vi "Set multiple channels.vi"(8 "values":dbl[](array[numeric]), 9 "names":string[](array[string]), 10 "Gateway IP Address (\"\": localhost)":string, 11 "Sequence Context":refnum<k7>) -> (0 "error out":errorcluster, 2 "Report Text":string)   [LabVIEW 2013, in "Set Channels.lvlib"]
uses:
  Set Channels.lvlib
  <vilib>/NI Veristand/Execution/Workspace/NI VeriStand - Set Multiple Channel Values.vi
  <vilib>/NI Veristand/Execution/Workspace/NI VeriStand - Get Multiple Channel Values.vi
  <vilib>/NI Veristand/Execution/Workspace/NI_VS Workspace ExecutionAPI.lvlib
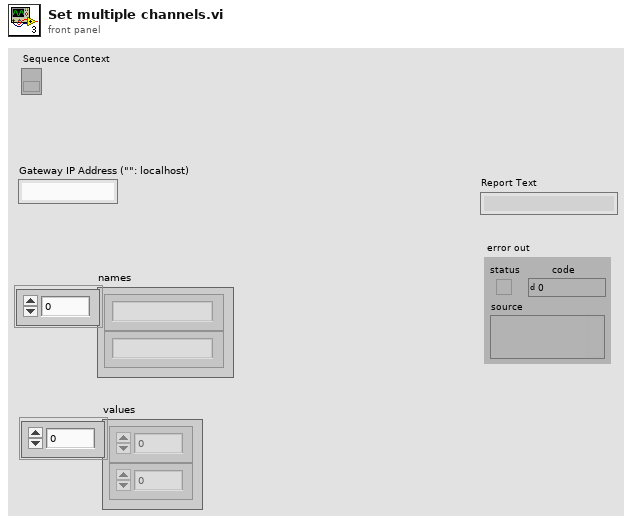
[diagram p1: front panel]
types:
  T1 = typedef "NI_VS Workspace ExecutionAPI.lvlib/WorkspaceAPI.ctl" = refnum<k24>
  T2 = typedef "TestStand - Status Monitor.ctl" = cluster{"Sequence Context":refnum<k7>, "Execution":refnum<k7>, "Termination Monitor":refnum<k7>}
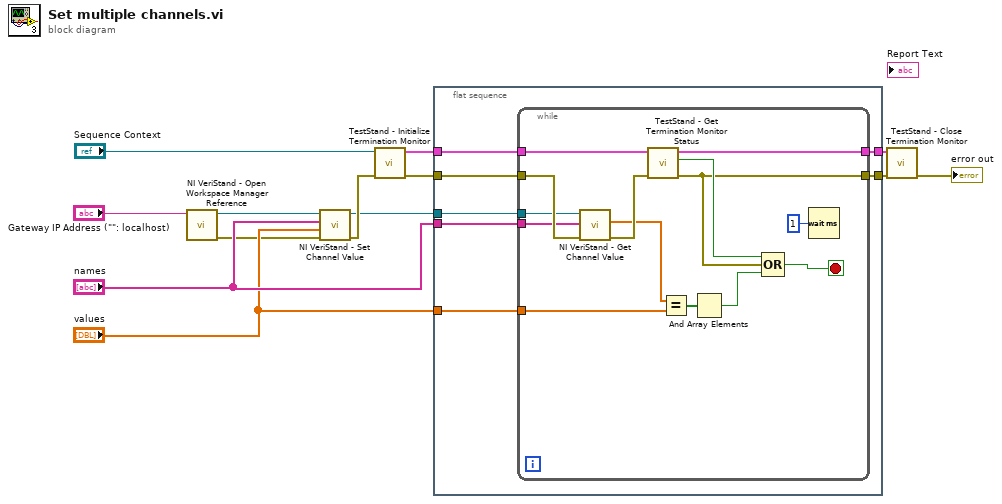
[diagram p0: block diagram]
diagram:
  n1 = call <vilib>:"NI VeriStand - Open Workspace Manager Reference.vi"("Gateway IP Address (\"\": localhost)"="Gateway IP Address (\"\": localhost)") -> ("error out"=w2:errorcluster, "WorkspaceManager"=w3:T1)  [unwired: 9 in]
  n2 = call-poly <vilib>:"NI VeriStand - Set Channel Value.vi"("error in (no error)"=w2, "Values"="values", "Channels"="names", "WorkspaceManager in"=w3) -> ("error out"=w13:errorcluster, "WorkspaceManager out"=w6:T1)  [unwired: 6 in]
  n3 = call <vilib>:"TestStand - Initialize Termination Monitor.vi"("error in (no error)"=w13, "Sequence Context In"="Sequence Context") -> ("error out"=w7:errorcluster, "Status Monitor Out"=w10:T2)  [unwired: 8 in]
  n4 = flat-sequence {
    tunnel: w10 -> [w20]
    tunnel: [w19] -> w9
    tunnel: [w18] -> w8
    tunnel: w7 -> [w17]
    tunnel: w6 -> [w16]
    tunnel: "names" -> [w15]
    tunnel: "values" -> [w14]
    frame #0 {
      n5 = while {
        tunnel: w20 -> [w30]
        tunnel: [w29] -> w19
        tunnel: [w28] -> w18
        tunnel: w17 -> [w26]
        tunnel: w16 -> [w25]
        tunnel: w15 -> [w24]
        tunnel: w14 -> [w23]
        stop <- w27 stop-if-true
        n6 = call-poly <vilib>:"NI VeriStand - Get Channel Value.vi"("error in (no error)"=w26, "Channels"=w24, "WorkspaceManager in"=w25) -> ("error out"=w34:errorcluster, "Values"=w33:dbl[])  [unwired: 6 in, 1 out]
        n7 = call <vilib>:"TestStand - Get Termination Monitor Status.vi"("error in (no error)"=w34, "Status Monitor In"=w30) -> ("error out"=w28:errorcluster, "Terminating or Aborting"=w32:bool, "Status Monitor Out"=w29:T2)  [unwired: 7 in]
        n8 = Equal?(x=w33, y=w23) -> (x = y?=w22:bool[])
        n9 = And Array Elements(Boolean array=w22) -> (logical AND=w21:bool)
        n10 = Compound Arithmetic op=OR(w32, w28, w21) -> (w27:bool)
        n11 = Wait (ms)(milliseconds to wait=u32 1) -> ()  [unwired: 1 out]
      }
    }
  }
  n12 = call <vilib>:"TestStand - Close Termination Monitor.vi"("error in (no error)"=w8, "Status Monitor In"=w9) -> ("error out"=→"error out":errorcluster)  [unwired: 9 in]
